vi "pyCode loginAuth.vi"(8 "error in (no error)":errorcluster, 10 "tokenFilePath":path, 11 "pyCode in":refnum<class "pyCode.lvclass">) -> (0 "error out":errorcluster, 3 "pyCode out":refnum<class "pyCode.lvclass">)   [LabVIEW 2018, in "pyCode.lvclass"]
uses:
  pyCode.lvclass
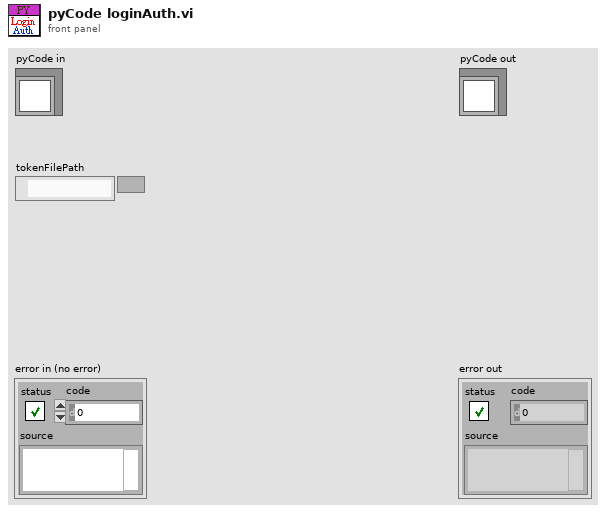
[diagram p1: front panel]
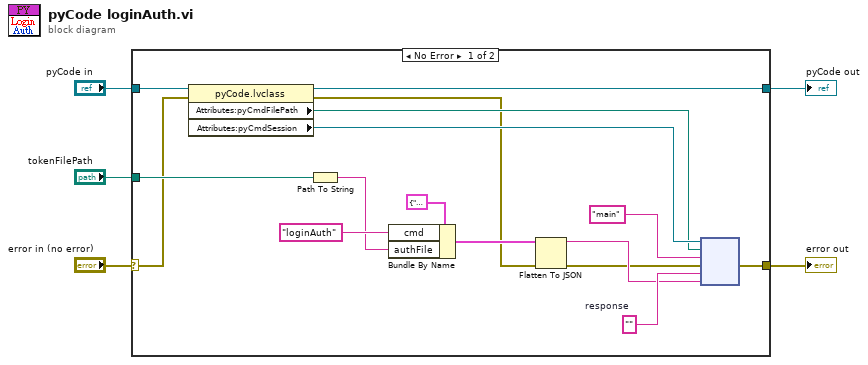
[diagram p0: block diagram]
diagram:
  n1 = case shown="No Error" "error in (no error)" {
    selector: "error in (no error)" -> [w8 w23]
    tunnel: [w6 w23] -> w4
    tunnel: [w20 w22] -> w2
    tunnel: "pyCode in" -> [w21 w22]
    tunnel: "tokenFilePath" -> [w11 _]
    frame No Error {
      w16 = ""  # response
      n2 = property class="pyCode.lvclass"(reference=w21, error in=w8) -> (reference out=w20:refnum<class "pyCode.lvclass">, error out=w7:errorcluster, "Attributes:pyCmdFilePath"=w18:path, "Attributes:pyCmdSession"=w19:refnum<k35>)
      n3 = Path To String(path=w11) -> (string=w13:string)
      n4 = Bundle By Name(cluster=cluster{"cmd":string, "authFile":string} {"cmd"="", "authFile"=""}, "cmd"="loginAuth", "authFile"=w13) -> (w12:cluster{"cmd":string, "authFile":string})
      n5 = Flatten To JSON(anything=w12, error in (no error)=w7) -> (JSON string=w10:string, 11:w9:errorcluster)  [unwired: 1 in]
      n6 = node(w19, w18, "main" ("function name"), w9, w16, w10) -> (w6:errorcluster)  [unwired: 2 in, 3 out]
    }
    frame Error {
    }
  }
  "error out" <- w4
  "pyCode out" <- w2
